vi "Function and Derivative.vi"(0 "result":dbl[](array[numeric]) format="%.2f", 1 "table":i32[][](array[numeric]), 2 "list of variables":i32[](array[numeric]), 3 "x":dbl=1e-08 format="%.2e", 4 "(x+h)-x":dbl=1e-08 format="%.2e") -> (5 "f(x)":dbl format="%.2f", 6 "df(x)/dx":dbl format="%.2f")   [LabVIEW 2014, in "NI_Gmath.lvlib"]
uses:
  NI_Gmath.lvlib
panel:
  # "operator"
  # "register1"
  # "register2"
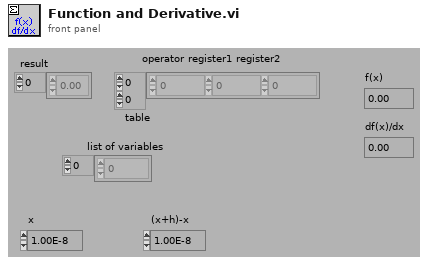
[diagram p1: front panel]
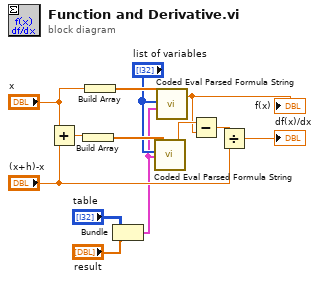
[diagram p0: block diagram]
diagram:
  n1 = Add(x="x", y="(x+h)-x") -> (x+y=w12:dbl)
  n2 = Build Array(w12) -> (w3:dbl[])
  n3 = Build Array("x") -> (w4:dbl[])
  n4 = Bundle("table"="table", "result"="result") -> (w1:cluster{"table":i32[][], "result":dbl[]})  [unwired: 1 in]
  n5 = call "Coded Eval Parsed Formula String.vi"("Parsed Formula"=w1, "Variables"="list of variables", "X Values"=w3) -> ("y value"=w11:dbl)  [unwired: 1 in, 1 out]
  n6 = call "Coded Eval Parsed Formula String.vi"("Parsed Formula"=w1, "Variables"="list of variables", "X Values"=w4) -> ("y value"=w10:dbl)  [unwired: 1 in, 1 out]
  "f(x)" <- w10
  n7 = Subtract(x=w11, y=w10) -> (x-y=w9:dbl)
  n8 = Divide(x=w9, y="(x+h)-x") -> (x/y=→"df(x)/dx":dbl)
